vi "曲线记录.vi"(7 "目录":string="HistoryData", 8 "基路径":path, 9 "检测序号":string="00000", 10 "YYYYMMDD":string, 11 "曲线数组":refnum<vi>[](array[refnum])) -> ()   [LabVIEW 2018]
uses:
  <vilib>/Utility/file.llb/Write Delimited Spreadsheet (DBL).vi
panel:
  out "路径":path
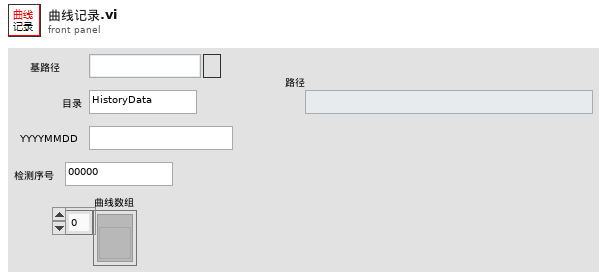
[diagram p1: front panel]
types:
  T1 = cluster{"力":sgl, "上限":sgl, "下限":sgl, "上参考":sgl, "下参考":sgl, "基准":sgl}[]
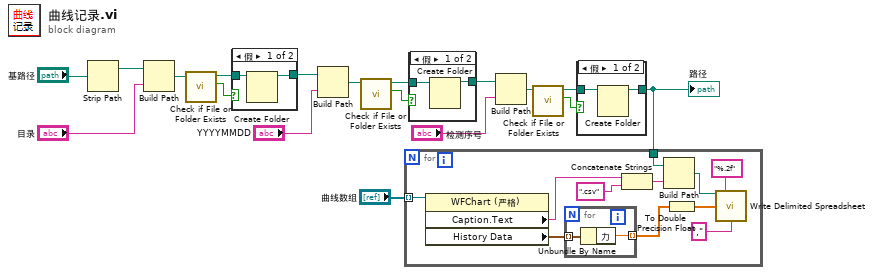
[diagram p0: block diagram]
diagram:
  n1 = Strip Path(path="基路径") -> (stripped path=w18:path)  [unwired: 1 out]
  n2 = Build Path(base path=w18, name or relative path="目录") -> (appended path=w9:path)
  n3 = call <vilib>:"Check if File or Folder Exists.vi"("path"=w9) -> ("file or folder exists?"=w7:bool, "dup path"=w8:path)  [unwired: 8 in, 1 out]
  n4 = case shown="假" w7 {
    tunnel: w8 -> [w20 w21]
    tunnel: [w19 w21] -> w6
    frame False {
      n5 = Create Folder(path (use dialog)=w20) -> (created path=w19:path)  [unwired: 2 in, 2 out]
    }
    frame True {
    }
  }
  n6 = Build Path(base path=w6, name or relative path="YYYYMMDD") -> (appended path=w17:path)
  n7 = call <vilib>:"Check if File or Folder Exists.vi"("path"=w17) -> ("file or folder exists?"=w16:bool, "dup path"=w15:path)  [unwired: 8 in, 1 out]
  n8 = case shown="假" w16 {
    tunnel: w15 -> [w23 w24]
    tunnel: [w22 w24] -> w14
    frame False {
      n9 = Create Folder(path (use dialog)=w23) -> (created path=w22:path)  [unwired: 2 in, 2 out]
    }
    frame True {
    }
  }
  n10 = Build Path(base path=w14, name or relative path="检测序号") -> (appended path=w13:path)
  n11 = call <vilib>:"Check if File or Folder Exists.vi"("path"=w13) -> ("file or folder exists?"=w12:bool, "dup path"=w11:path)  [unwired: 8 in, 1 out]
  n12 = case shown="假" w12 {
    tunnel: w11 -> [w26 w27]
    tunnel: [w25 w27] -> w5
    frame False {
      n13 = Create Folder(path (use dialog)=w26) -> (created path=w25:path)  [unwired: 2 in, 2 out]
    }
    frame True {
    }
  }
  "路径" <- w5
  n14 = for {
    tunnel: "曲线数组" -> [w33] mode=indexing
    tunnel: w5 -> [w31]
    n15 = property class="WFChart (严格)"(reference=w33) -> ("Caption.Text"=w32:string, "History Data"=w30:T1)  [unwired: 1 in, 2 out]
    n16 = for {
      tunnel: w30 -> [w40] mode=indexing
      tunnel: [w39] -> w28 mode=indexing
      n17 = Unbundle By Name(w40) -> ("力"=w39:sgl)
    }
    n18 = Concatenate Strings(w32, ".csv" ("字符串")) -> (w35:string)
    n19 = Build Path(base path=w31, name or relative path=w35) -> (appended path=w36:path)
    n20 = To Double Precision Float(number=w28) -> (double precision float=w29:dbl[])
    n21 = call-poly <vilib>:"Write Delimited Spreadsheet.vi"("file path (dialog if empty)"=w36, "format (%.3f)"="%.2f", "1D data"=w29, "delimiter (\\t)"="," ("delimiter (\\t)")) -> ()  [unwired: 10 in, 2 out]
  }
